vi "_FPGA_Driver_AD5648_v1.4.vi"(6 "Cmd#":u8, 8 "AO Data":u16, 9 "Channel#":u8, 10 "Update_latch":bool) -> (2 "Updating?":bool)   [LabVIEW 2018]
uses:
  <vilib>/rvi/eio/common/nirviEmuTemplateMethod_errors.vi
  <vilib>/eio/EIONode/EIONode.xnode
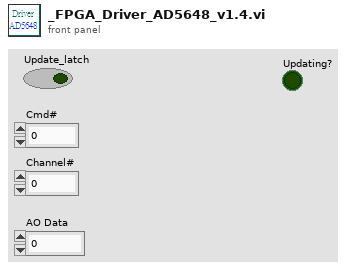
[diagram p1: front panel]
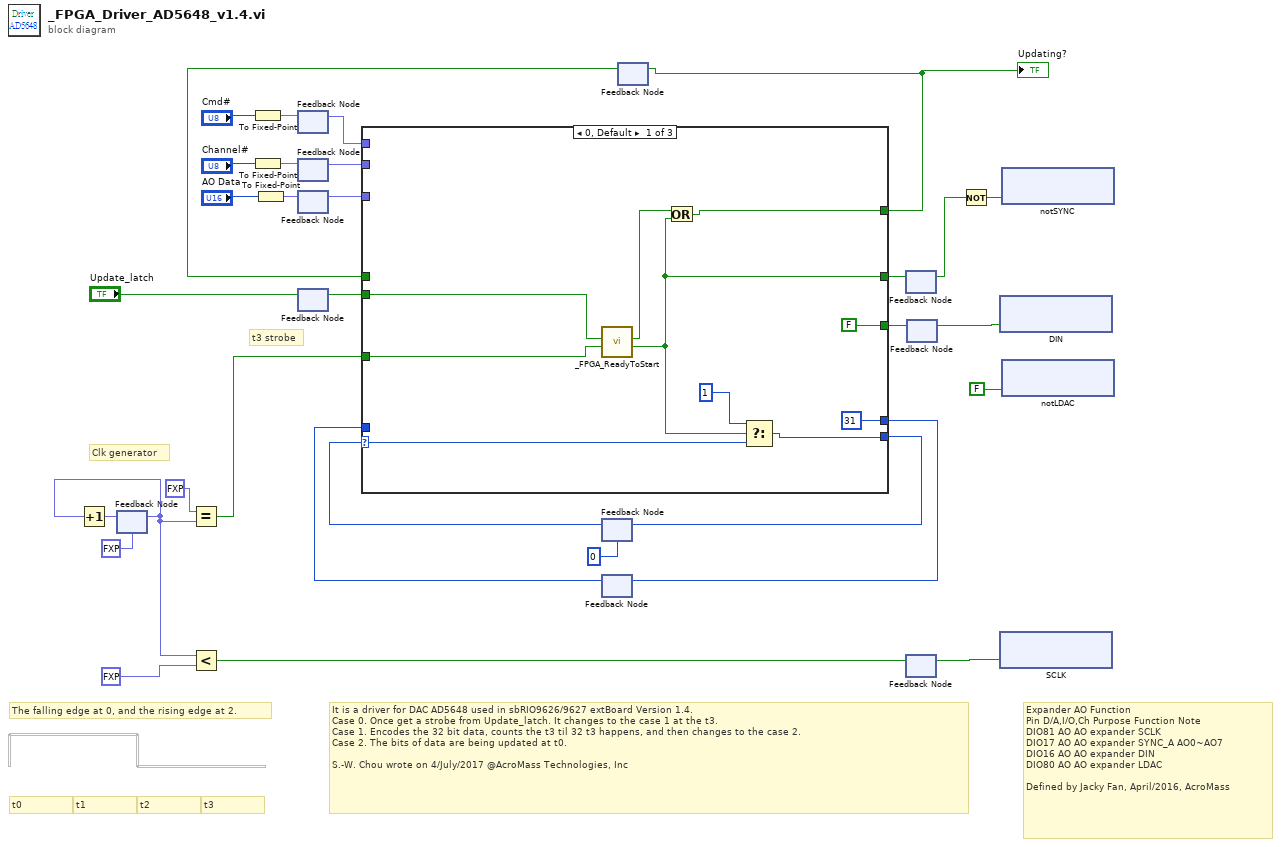
[diagram p0: block diagram]
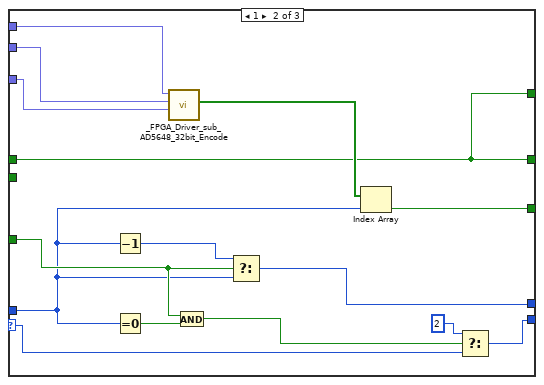
[diagram p2: hidden frame]
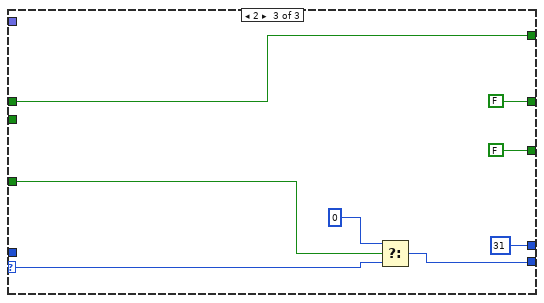
[diagram p3: hidden frame]
diagram:
  # "t3 strobe"
  # "Clk generator"
  # "It is a driver for DAC AD5648 used in sbRIO9626/9627 extBoard Version 1.4.\nCase 0. Once get a strobe from Update_latch. It changes to the case 1 at the t3.\nCase 1. Encodes the 32 bit data, counts the t3 til 32 t3 happens, and then changes to the case 2.\nCase 2. The bits of data are being updated at t0.\n\nS.-W. Chou wrote on 4/July/2017 @AcroMass Technologies, Inc"
  # "t3"
  # "t2"
  # "t1"
  # "t0"
  # "The falling edge at 0, and the rising edge at 2."
  # "Expander AO Function\t\t\t\t\nPin\tD/A,I/O,Ch\tPurpose\tFunction\tNote\nDIO81\tAO\tAO expander\tSCLK\t\nDIO17\tAO\tAO expander\tSYNC_A\tAO0~AO7\nDIO16\tAO\tAO expander\tDIN\t\nDIO80\tAO\tAO expander\tLDAC\t\n\nDefined by Jacky Fan, April/2016, AcroMass"
  n1 = feedback #1(fxp<+,2,2> 0.0) -> (w18:fxp<+,2,2>)
  n2 = Increment(x=w18) -> (x+1=w20:fxp<+,2,2>)
  n3 = feedback-in #1(w20) -> ()
  n4 = Equal?(x=fxp<+,2,2> 3.0, y=w18) -> (x = y?=w3:bool)
  n5 = Less?(x=w18, y=fxp<+,2,2> 2.0) -> (x < y?=w16:bool)
  n6 = To Fixed-Point(number="Cmd#") -> (fixed-point=w11:fxp<+,4,4>)  [unwired: 1 in]
  n7 = To Fixed-Point(number="Channel#") -> (fixed-point=w25:fxp<+,4,4>)  [unwired: 1 in]
  n8 = To Fixed-Point(number="AO Data") -> (fixed-point=w27:fxp<+,14,14>)  [unwired: 1 in]
  n9 = feedback #2() -> (w9:fxp<+,4,4>)  [unwired: 1 in]
  n10 = feedback-in #2(w11) -> ()
  n11 = feedback-in #3(w25) -> ()
  n12 = feedback #3() -> (w29:fxp<+,4,4>)  [unwired: 1 in]
  n13 = feedback #4() -> (w28:fxp<+,14,14>)  [unwired: 1 in]
  n14 = feedback-in #4(w27) -> ()
  n15 = feedback-in #5("Update_latch") -> ()
  n16 = feedback #5() -> (w14:bool)  [unwired: 1 in]
  n17 = feedback #6(u8 0) -> (w31:u8)
  n18 = feedback #7() -> (w22:u8)  [unwired: 1 in]
  n19 = feedback #8() -> (w2:bool)  [unwired: 1 in]
  n20 = case shown="0, Default" w31 {
    selector: w31 -> [w41 w54 w60]
    tunnel: w2 -> [_ w43 w58]
    tunnel: [w39 w52 w61] -> w15
    tunnel: w29 -> [_ w48 _]
    tunnel: w28 -> [_ w47 _]
    tunnel: w3 -> [w36 w50 w63]
    tunnel: [FALSE w49 FALSE] -> w24
    tunnel: [u8 31 w56 u8 31] -> w23
    tunnel: w22 -> [_ w45 _]
    tunnel: w14 -> [w38 _ _]
    tunnel: [w33 w43 FALSE ("Ready?")] -> w13
    tunnel: w9 -> [_ w44 _]
    tunnel: [w34 w43 w58] -> w1
    frame 0, Default {
      n21 = call "_FPGA_ReadyToStart.vi"("Start_strobe_in"=w36, "Ready_latch_in"=w38) -> ("Trigger_strobe_out"=w33:bool, "Ready?"=w35:bool)  [unwired: 8 in]
      n22 = Or(x=w35, y=w33) -> (x .or. y?=w34:bool)
      n23 = Select(t=u8 1, s=w33, f=w41) -> (s? t:f=w39:u8)
    }
    frame 1 {
      n24 = Decrement(x=w45) -> (x-1=w57:u8)
      n25 = Equal To 0?(x=w45) -> (x = 0?=w55:bool)
      n26 = call "_FPGA_Driver_sub_AD5648_32bit_Encode.vi"("data_U14"=w47, "address_U4"=w48, "cmd"=w44) -> ("Data_out"=w46:bool[])  [unwired: 8 in]
      n27 = And(x=w50, y=w55) -> (x .and. y?=w51:bool)
      n28 = Select(t=w57, s=w50, f=w45) -> (s? t:f=w56:u8)
      n29 = Index Array(array=w46, index=w45) -> (element=w49:bool)
      n30 = Select(t=u8 2, s=w51, f=w54) -> (s? t:f=w52:u8)
    }
    frame 2 {
      n31 = Select(t=u8 0, s=w63, f=w60) -> (s? t:f=w61:u8)
    }
  }
  "Updating?" <- w1
  n32 = feedback-in #6(w15) -> ()
  n33 = feedback-in #7(w23) -> ()
  n34 = feedback-in #8(w1) -> ()
  n35 = feedback #9() -> (w5:bool)  [unwired: 1 in]
  n36 = feedback-in #9(w13) -> ()
  n37 = feedback-in #10(w16) -> ()
  n38 = feedback #10() -> (w8:bool)  [unwired: 1 in]
  n39 = feedback-in #11(w24) -> ()
  n40 = feedback #11() -> (w6:bool)  [unwired: 1 in]
  n41 = Not(x=w5) -> (.not. x?=w7:bool)
  n42 = xnode "DIN"("RMC/DIO16"=w6) -> ()  [unwired: 1 in, 1 out]
  n43 = xnode "SCLK"("RMC/DIO81"=w8) -> ()  [unwired: 1 in, 1 out]
  n44 = xnode "notSYNC"("RMC/DIO17"=w7) -> ()  [unwired: 1 in, 1 out]
  n45 = xnode "notLDAC"("RMC/DIO80"=FALSE) -> ()  [unwired: 1 in, 1 out]
